vi "UNIT_TEST_TEMPLATE.vi"(8 "error in (no error)":errorcluster, 11 "TestObservation In":refnum<class "TestObservation.lvclass">) -> (0 "error out":errorcluster, 3 "TestObservation Out":refnum<class "TestObservation.lvclass">)   [LabVIEW 2015, in "TestObservation.lvclass"]
uses:
  TestObservation.lvclass
  <vilib>/addons/_JKI Toolkits/VI Tester/TestCase.llb/TestCase.lvclass
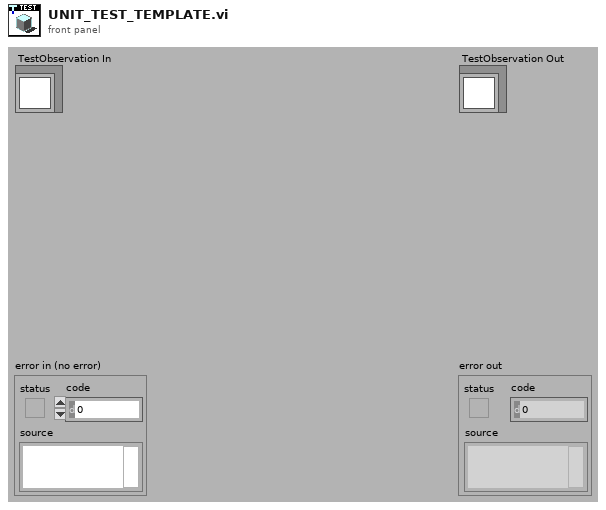
[diagram p1: front panel]
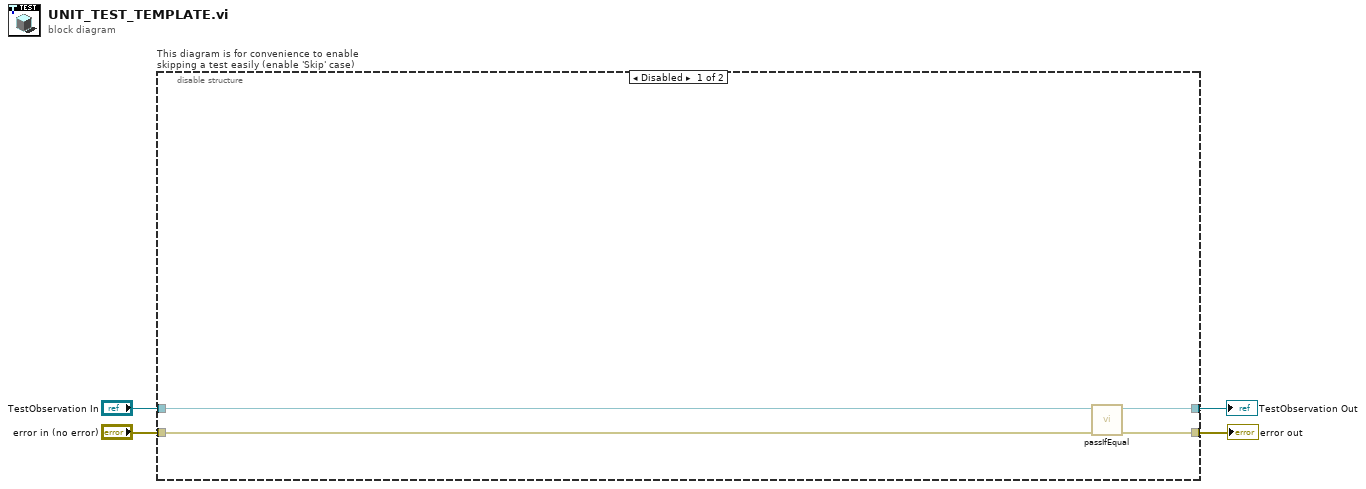
[diagram p0: block diagram]
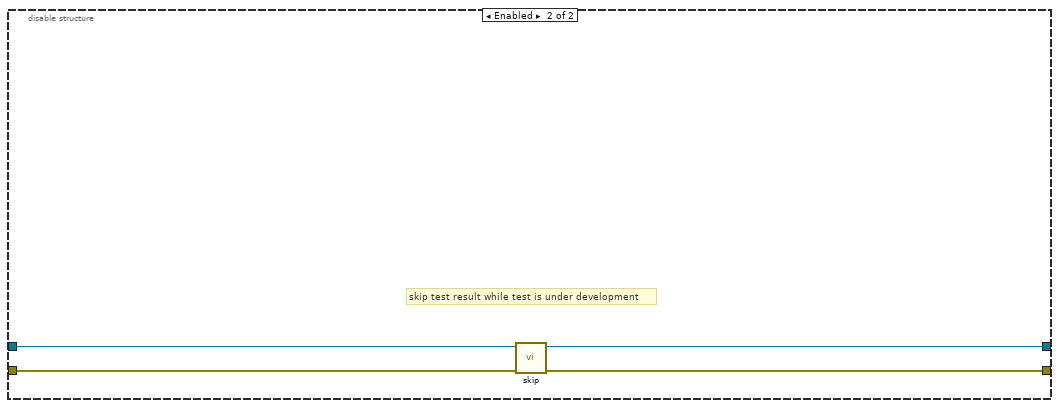
[diagram p2: hidden frame]
diagram:
  n1 = disable-structure "This diagram is for convenience to enable skipping a test easily (enable 'Skip' case)" shown="Disabled" {
    disable-tunnel: "TestObservation In" -> [w8 w12]
    disable-tunnel: [w7 w10] -> w1
    disable-tunnel: [w6 w11] -> w3
    disable-tunnel: "error in (no error)" -> [w5 w9]
    frame Disabled {
      n2 = call-dynamic "passIfEqual.vi"("error in (no error)"=w5, "TestCase in"=w8) -> ("error out"=w6:errorcluster, "TestCase out"=w7:refnum<class "TestObservation.lvclass">)  [unwired: 8 in]
    }
    frame Enabled {
      # "skip test result while test is under development"
      n3 = call <vilib>:"skip.vi"("error in (no error)"=w9, "TestCase in"=w12) -> ("error out"=w11:errorcluster, "TestCase out"=w10:refnum<class "TestObservation.lvclass">)  [unwired: 8 in]
    }
  }
  "error out" <- w3
  "TestObservation Out" <- w1
